vi "GUI_HTU_control.vi"() -> ()   [LabVIEW 2013]
uses:
  shared programs/GUI_Template/GUI_master/tcp_new_data_event.ctl
  shared programs/GUI_Template/GUI_master/tcp new data cluster.ctl
panel:
  in  "pos.Channel1::9":enum16{"1", "2", "3", "4", "5", "6"}(ring) caption="Garting Mode filter"
  in  "GUIdevice 9":string="U_FilterwheelGratingMode"
  in  "pos.Channel3::5":enum16{"1", "2", "3", "4", "5", "6"}(ring) caption="Phasics"
  in  "pos.Channel2::5":enum16{"1", "2", "3", "4", "5", "6"}(ring) caption="Ghost pulsed"
  in  "pos.Channel1::5":enum16{"1", "2", "3", "4", "5", "6"}(ring) caption="StellarNet Spectrometer"
  in  "AnalogOutput.Channel 1::8":dbl caption="PressureControlVoltage" min=0.0 max=3.0
  in  "Position.Axis 3::7":dbl caption="Jet_Z" min=0.0 max=25.0
  in  "Position.Axis 2::7":dbl caption="Jet_Y" min=-25.0 max=0.0
  in  "Position.Axis 1::7":dbl caption="Jet_X" min=0.0 max=25.0
  in  "GUIdevice 8":string="U_HP_Daq"
  in  "GUIdevice 7":string="U_ESP_JetXYZ"
  in  "pos.Channel0::5":enum16{"1", "2", "3", "4", "5", "6"}(ring) caption="Mode Imager Filter"
  in  "Position.Channel 2::2":T1(ring) caption="Beamline In"
  in  "Position.Channel 1::2":T1(ring) caption="Beamline Out"
  in  "Position.Channel 6::1":T1(ring) caption="Gaia Beamblock 3-North"
  in  "Position.Channel 5::1":T1(ring) caption="Gaia Beamblock 4-North"
  in  "Position.Channel 4::1":T1(ring) caption="Gaia Stop South"
  in  "Position.Channel 3::1":T1(ring) caption="Gaia Stop North"
  in  "Position.Channel 2::1":T1(ring) caption="Gaia Beamblock 3-South"
  in  "Position.Channel 1::1":T1(ring) caption="Gaia Beamblock 4-South"
  in  "Position.Axis 1::6":dbl caption="Mode Imager Position" min=-60.0 max=20.0
  in  "GUIdevice 6":string="U_ModeImagerESP"
  in  "GUIdevice 5":string="U_FilterWheel_01"
  in  "Position.Axis 6::4":dbl caption="Beamline In Y" min=0.0 max=6.0
  in  "Position.Axis 5::4":dbl caption="Beamline In X" min=0.0 max=6.0
  in  "Position.Axis 4::4":dbl caption="Beamline Out Y" min=0.0 max=6.0
  in  "Position.Axis 3::4":dbl caption="Beamline Out X" min=0.0 max=6.0
  in  "Position.Axis 2::4":dbl caption="OAP In 2 Y" min=0.0 max=6.0
  in  "Position.Axis 1::4":dbl caption="OAP In 2 X" min=0.0 max=6.0
  in  "Position.Axis 6::3":dbl caption="OAP In 1 Y" min=0.0 max=6.0
  in  "Position.Axis 5::3":dbl caption="OAP In 1 X" min=0.0 max=6.0
  in  "Position.Axis 4::3":dbl caption="Comp In Y" min=0.0 max=6.0
  in  "Position.Axis 3::3":dbl caption="Comp In X" min=0.0 max=6.0
  in  "Position.Axis 2::3":dbl caption="Tube In Y" min=0.0 max=6.0
  in  "Position.Axis 1::3":dbl caption="Tube In X" min=0.0 max=6.0
  in  "GUIdevice 4":string="U_TRAServer02"
  in  "GUIdevice 3":string="U_TRAServer01"
  in  "GUIdevice 2":string="U_1Wire_Bcave"
  out "tcp data event":T2
  out "error IO 2":errorcluster
  in  "GUIdevice 1":string="U_1Wire_148"
  in  "?":bool
  # "Room 148"
  # "B-Cave"
  # "Flippers"
  # "XHairs"
  # "Gas Jet"
  # "Mode Imager"
  # "TRA motors"
  # "TRA motors"
  # "Pressure controller"
  # "Filter Wheels"
  # "Filter wheel grating mode"
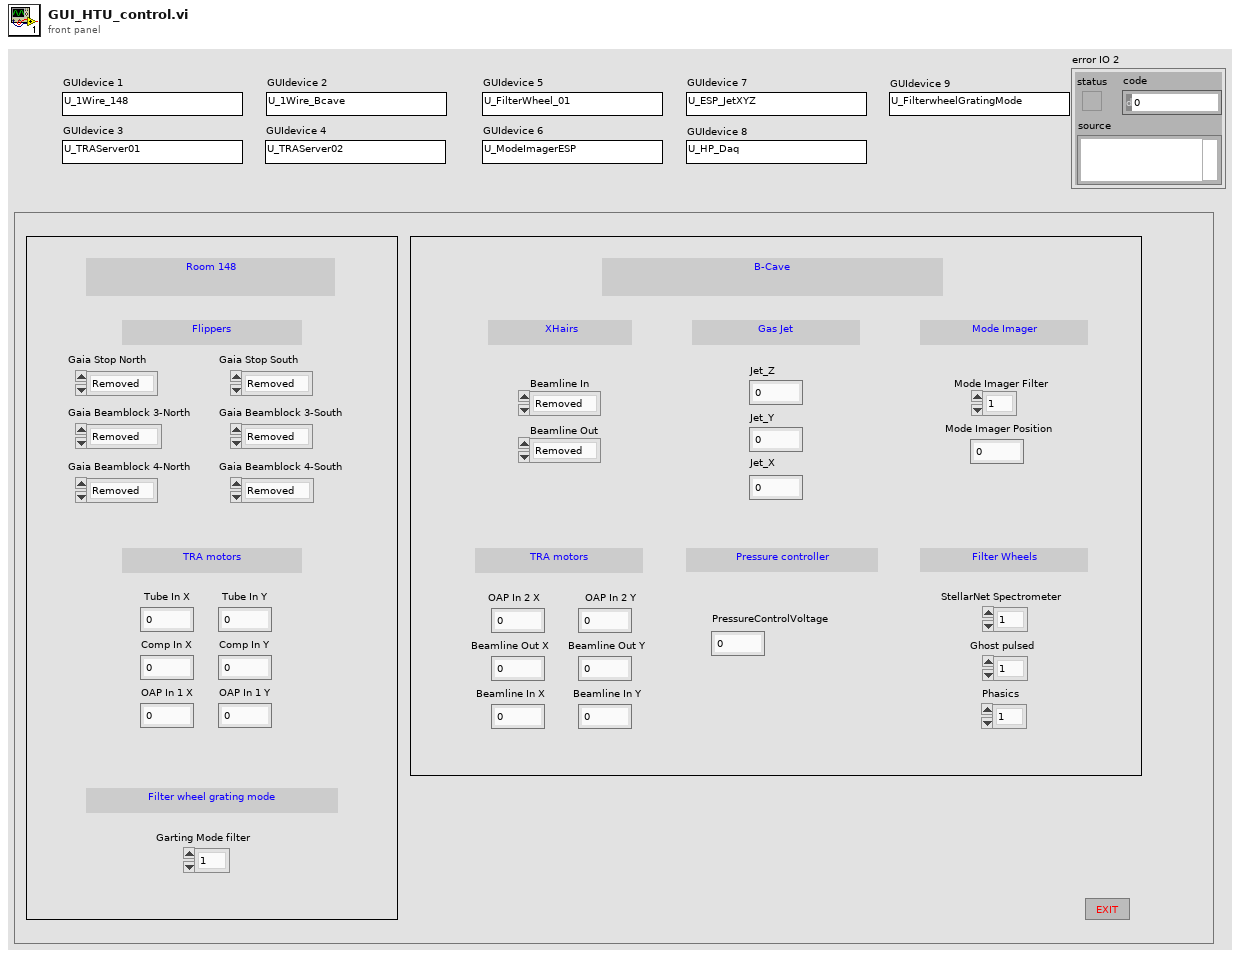
[diagram p1: front panel]
types:
  T1 = enum16{"Removed", "Inserted", "Unknown", "Moving"}
  T2 = typedef "tcp_new_data_event.ctl" = refnum<user-event>
  T3 = typedef "tcp new data cluster.ctl" = cluster{"EventEnum":enum16{"new data", "connection status update"}, "Device name":string}
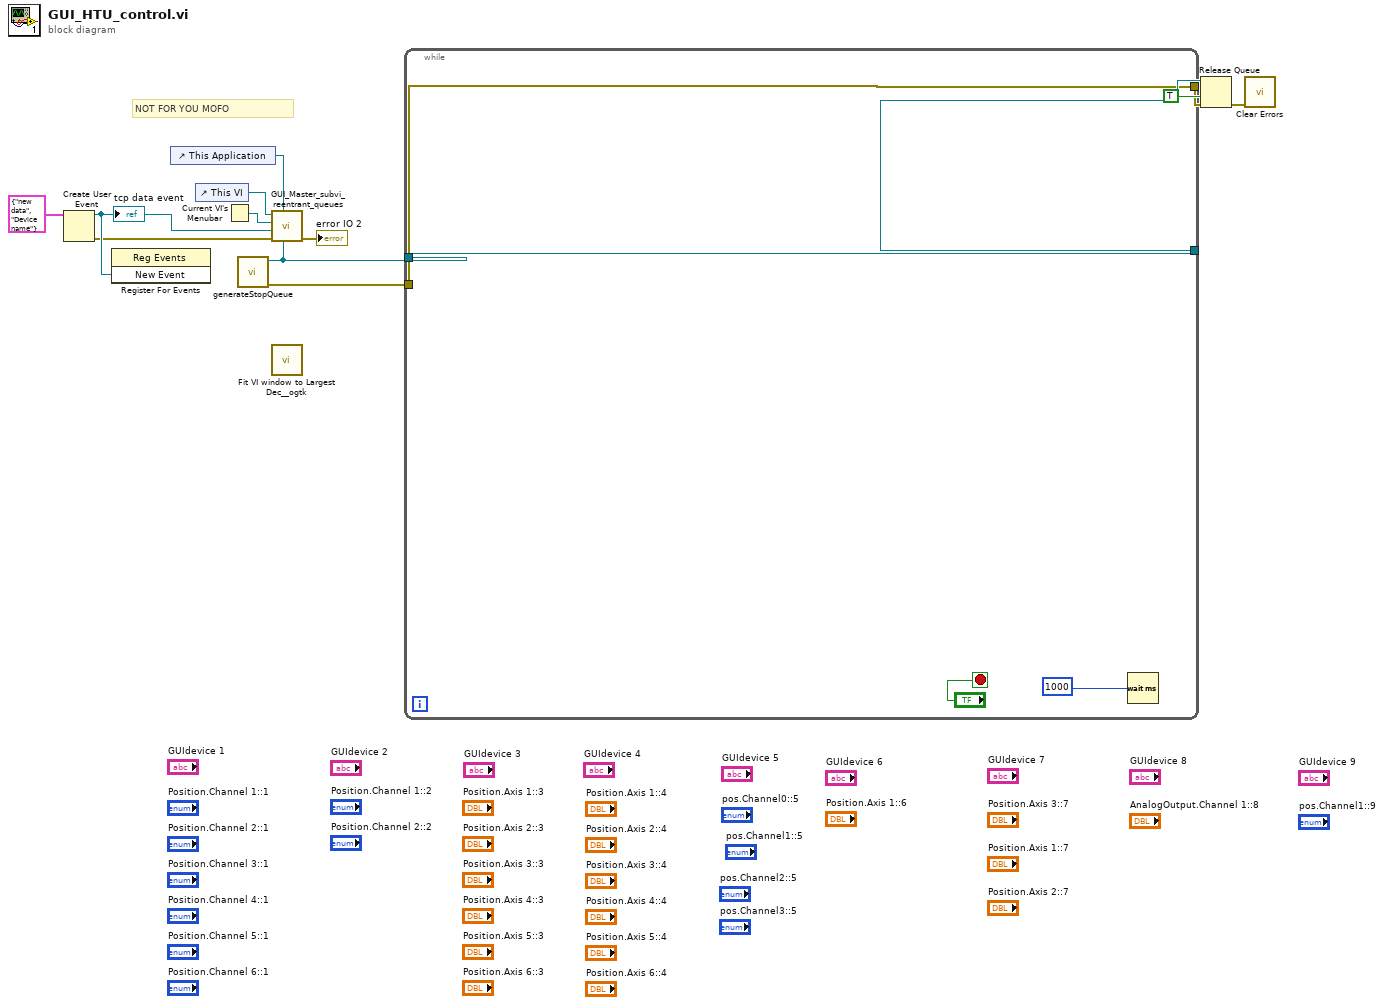
[diagram p0: block diagram]
diagram:
  # "NOT FOR YOU MOFO"
  n1 = Create User Event(user event datatype=T3 {"EventEnum"=enum."new data", "Device name"="Device name"} ("New Event")) -> (user event=w8:refnum<user-event>, error out=w7:errorcluster)  [unwired: 1 in]
  "tcp data event" <- w8
  n2 = register-events(w8) -> ()  [unwired: 2 in, 2 out]
  n3 = control-ref of="This Application"() -> (w9:refnum<vi>)
  n4 = control-ref of="This VI"() -> (w4:refnum<vi>)
  n5 = Current VI's Menubar() -> (w5:refnum<k9>)
  n6 = call "generateStopQueue.vi"() -> ("error out"=w2:errorcluster, "STOP Queue out"=w1:refnum<queue>)  [unwired: 10 in]
  n7 = call "GUI_Master_subvi_reentrant_queues.vi"("STOP Queue in"=w1, "This Application"=w9, "error in (no error)"=w7, "tcp data event"=w8, "Caller menu reference"=w5, "Caller VI ref"=w4) -> ("error out"=→"error IO 2":errorcluster)  [unwired: 5 in]
  n8 = call <userlib>:"Fit VI window to Largest Dec__ogtk.vi"() -> ()  [unwired: 6 in, 2 out]
  n9 = while {
    tunnel: [w16] -> w11
    tunnel: w2 -> [w16]
    tunnel: w1 -> [w15]
    tunnel: [w15] -> w10
    stop <- "?" stop-if-true
    n10 = Wait (ms)(milliseconds to wait=u32 1000) -> ()  [unwired: 1 out]
  }
  n11 = Release Queue(queue=w10, force destroy? (F)=TRUE, error in (no error)=w11) -> (error out=w13:errorcluster)  [unwired: 2 out]
  n12 = call <vilib>:"Clear Errors.vi"("error in (no error)"=w13) -> ()  [unwired: 6 in, 1 out]
